vi "AMI MAG PHI IS_temp.vi"(0 "Y-Axis Communications Config":T3, 1 "delta H (mT)":dbl=0.5, 2 "delta phi (deg)":dbl=0.5, 3 "sweep parameter":T1=enum."magnetic field", 4 "const phi?":bool, 5 "Z-Axis Communications Config":T3, 7 "target mag in (T)":dbl, 9 "target phi (deg)":dbl, 11 "error in (no error)":T2) -> (6 "target mag out (T)":dbl[](array[numeric]), 8 "phi array (deg)":dbl[](array[numeric]), 15 "error out":T2)   [LabVIEW 2013]
uses:
  measurement/measurement sweep parameter.ctl
  <vilib>/Analysis/1siggen.llb/Ramp Pattern by Delta.vi
  <vilib>/Analysis/NI_AALBase.lvlib
panel:
  out "current mag (kG)":dbl
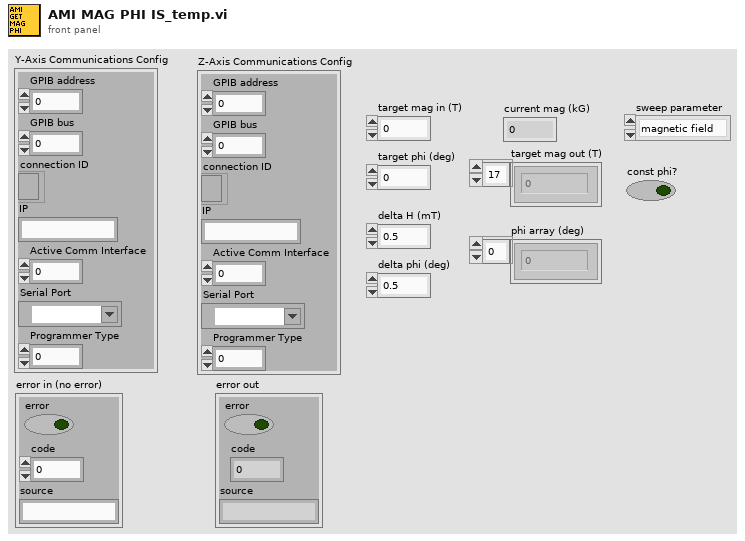
[diagram p1: front panel]
types:
  T1 = typedef "measurement sweep parameter.ctl" = enum16{"angle", "magnetic field"}
  T2 = cluster{"error":bool, "code":i32, "source":string}
  T3 = cluster{"GPIB address":i16, "GPIB bus":i16, "connection ID":refnum<k5>, "IP":string, "Active Comm Interface":u16, "Serial Port":refnum<visa-resource-name>, "Programmer Type":u16}
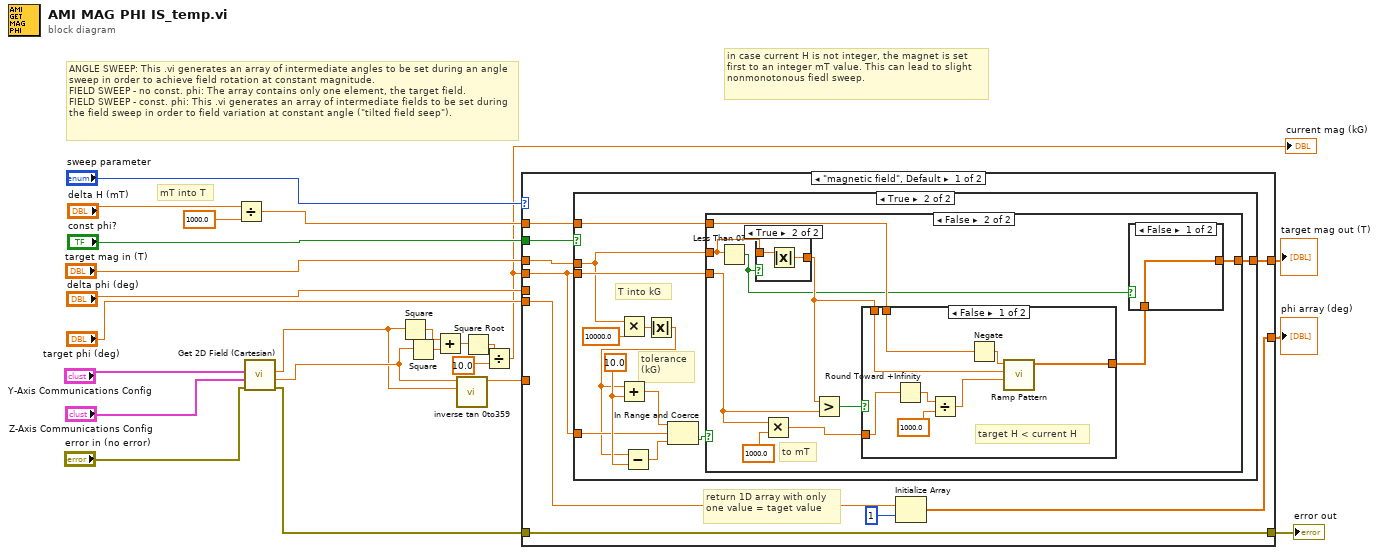
[diagram p0: block diagram]
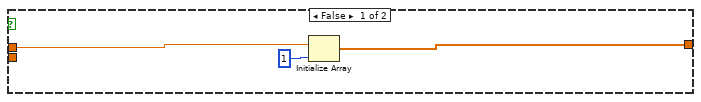
[diagram p2: hidden frame]
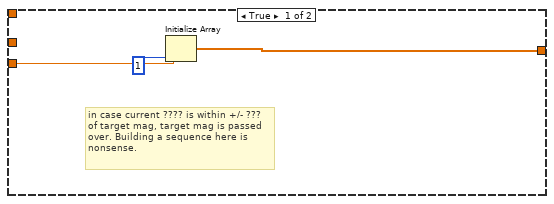
[diagram p3: hidden frame]
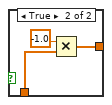
[diagram p4: hidden frame]
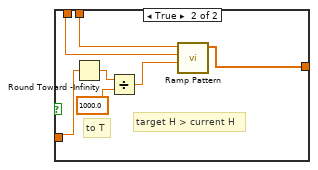
[diagram p6: hidden frame]
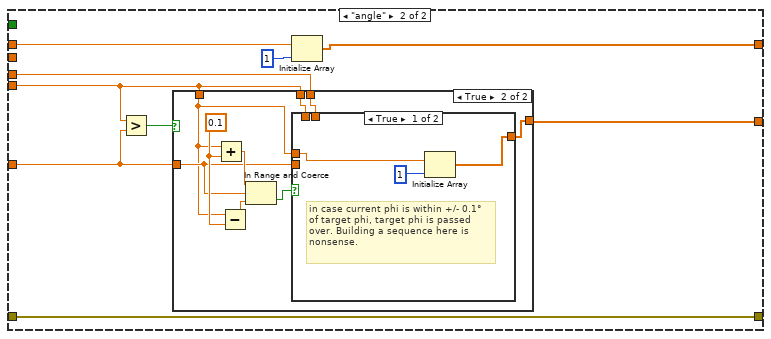
[diagram p7: hidden frame]
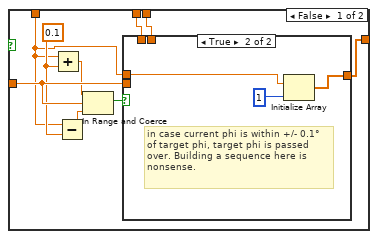
[diagram p8: hidden frame]
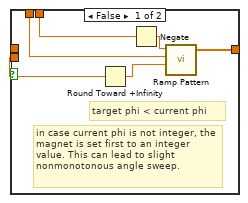
[diagram p9: hidden frame]
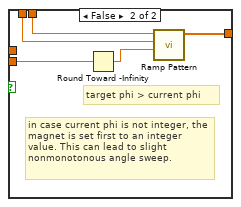
[diagram p10: hidden frame]
diagram:
  # "in case current H is not integer, the magnet is set first to an integer mT value. This can lead to slight nonmonotonous fiedl sweep."
  # "mT into T"
  # "ANGLE SWEEP: This .vi generates an array of intermediate angles to be set during an angle sweep in order to achieve field rotation at constant magnitude.\nFIELD SWEEP - no const. phi: The array contains only one element, the target field.\nFIELD SWEEP - const. phi: This .vi generates an array of intermediate fields to be set during the field sweep in order to field variation at constant angle (\"tilted field seep\")."
  n1 = Divide(x="delta H (mT)", y=1000.0) -> (x/y=w5:dbl)
  n2 = call <userlib>:"Get 2D Field (Cartesian).vi"("Y-Axis Communications Config"="Y-Axis Communications Config", "Z-Axis Communications Config"="Z-Axis Communications Config", "error in"="error in (no error)") -> ("Y-Axis Field (kG)"=w9:dbl, "Z-Axis Field (kG)"=w10:dbl, "error out"=w12:T2)  [unwired: 2 in, 1 out]
  n3 = Square(x=w9) -> (x^2=w20:dbl)
  n4 = Square(x=w10) -> (x^2=w19:dbl)
  n5 = Add(x=w20, y=w19) -> (x+y=w21:dbl)
  n6 = call "inverse tan 0to359.vi"("y coil"=w9, "z coil"=w10) -> ("phi (deg)"=w11:dbl)  [unwired: 9 in]
  n7 = Square Root(x=w21) -> (sqrt(x)=w1:dbl)
  n8 = Divide(x=w1, y=10.0) -> (x/y=w3:dbl)
  "current mag (kG)" <- w3
  n9 = case shown="\"magnetic field\", Default" "sweep parameter" {
    tunnel: "target phi (deg)" -> [w30 w84]
    tunnel: w11 -> [_ w88]
    tunnel: "delta phi (deg)" -> [_ w92]
    tunnel: [w31 w91] -> w16
    tunnel: [w28 w85] -> w8
    tunnel: "target mag in (T)" -> [w29 w86]
    tunnel: [w32 w90] -> w13
    tunnel: w12 -> [w32 w90]
    tunnel: "const phi?" -> [w27 _]
    tunnel: w3 -> [w25 _]
    tunnel: w5 -> [w26 _]
    frame "magnetic field", Default {
      # "return 1D array with only one value = taget value"
      n10 = case shown="True" w27 {
        tunnel: w29 -> [w35 w40]
        tunnel: [w34 w48] -> w28
        tunnel: w25 -> [_ w47]
        tunnel: w26 -> [_ w37]
        tunnel: w25 -> [_ w42]
        frame False {
          n11 = Initialize Array(w35, 1) -> (w34:dbl[])
        }
        frame True {
          w46 = 10.0
          # "tolerance (kG)"
          # "T into kG"
          n12 = Multiply(x=w40, y=10000.0) -> (x*y=w39:dbl)
          n13 = Absolute Value(x=w39) -> (abs(x)=w38:dbl)
          n14 = Add(x=w38, y=w46) -> (x+y=w44:dbl)
          n15 = Subtract(x=w38, y=w46) -> (x-y=w45:dbl)
          n16 = In Range and Coerce(upper limit=w44, x=w42, lower limit=w45) -> (In Range?=w43:bool)  [unwired: 1 out]
          n17 = case shown="False" w43 {
            tunnel: w40 -> [_ w55]
            tunnel: [w50 w52] -> w48
            tunnel: w47 -> [w49 w56]
            tunnel: w37 -> [_ w57]
            frame True {
              # "in case current ???? is within +/- ??? of target mag, target mag is passed over. Building a sequence here is nonsense."
              n18 = Initialize Array(w49, 1) -> (w50:dbl[])
            }
            frame False {
              # "to mT"
              n19 = Less Than 0?(x=w55) -> (x < 0?=w54:bool)
              n20 = case shown="True" w54 {
                tunnel: w55 -> [w66 w68]
                tunnel: [w66 w67] -> w58
                frame False {
                }
                frame True {
                  n21 = Absolute Value(x=w68) -> (abs(x)=w67:dbl)
                }
              }
              n22 = Multiply(x=w56, y=1000.0) -> (x*y=w60:dbl)
              n23 = Greater?(x=w58, y=w56) -> (0:w61:bool)
              n24 = case shown="False" w61 {
                tunnel: w58 -> [w74 w83]
                tunnel: w60 -> [w69 w77]
                tunnel: w57 -> [w75 w82]
                tunnel: [w73 w81] -> w53
                frame False {
                  # "target H < current H"
                  n25 = Round Toward +Infinity(x=w69) -> (ceil(x): smallest int >= x=w72:dbl)
                  n26 = Divide(x=w72, y=1000.0) -> (x/y=w70:dbl)
                  n27 = Negate(x=w75) -> (-x=w76:dbl)
                  n28 = call-poly <vilib>:"Ramp Pattern.vi"("start"=w70, "end"=w74, "delta"=w76) -> ("Ramp Pattern"=w73:dbl[])  [unwired: 6 in, 2 out]
                }
                frame True {
                  # "to T"
                  # "target H > current H"
                  n29 = Round Toward -Infinity(1:w77) -> (0:w80:dbl)
                  n30 = Divide(x=w80, y=1000.0) -> (x/y=w78:dbl)
                  n31 = call-poly <vilib>:"Ramp Pattern.vi"("start"=w78, "end"=w83, "delta"=w82) -> ("Ramp Pattern"=w81:dbl[])  [unwired: 6 in, 2 out]
                }
              }
              n32 = case shown="False" w54 {
                tunnel: w53 -> [w62 w64]
                tunnel: [w62 w63] -> w52
                frame False {
                }
                frame True {
                  n33 = Multiply(x=-1.0, y=w64) -> (x*y=w63:dbl[])
                }
              }
            }
          }
        }
      }
      n34 = Initialize Array(w30, 1) -> (w31:dbl[])
    }
    frame "angle" {
      n35 = Greater?(x=w84, y=w88) -> (0:w89:bool)
      n36 = case shown="True" w89 {
        tunnel: w84 -> [w100 w119]
        tunnel: w88 -> [w97 w112]
        tunnel: w92 -> [w101 w118]
        tunnel: [w99 w117] -> w91
        tunnel: w84 -> [w93 w111]
        frame False {
          w94 = 0.1
          n37 = Add(x=w93, y=w94) -> (x+y=w96:dbl)
          n38 = Subtract(x=w93, y=w94) -> (x-y=w95:dbl)
          n39 = In Range and Coerce(upper limit=w96, x=w97, lower limit=w95) -> (In Range?=w98:bool)  [unwired: 1 out]
          n40 = case shown="True" w98 {
            tunnel: w97 -> [w103 _]
            tunnel: w101 -> [w104 _]
            tunnel: w100 -> [w102 _]
            tunnel: [w105 w110] -> w99
            tunnel: w93 -> [_ w108]
            frame False {
              # "in case current phi is not integer, the magnet is set first to an integer value. This can lead to slight nonmonotonous angle sweep."
              # "target phi < current phi"
              n41 = Round Toward +Infinity(x=w103) -> (ceil(x): smallest int >= x=w107:dbl)
              n42 = Negate(x=w104) -> (-x=w106:dbl)
              n43 = call-poly <vilib>:"Ramp Pattern.vi"("start"=w107, "end"=w102, "delta"=w106) -> ("Ramp Pattern"=w105:dbl[])  [unwired: 6 in, 2 out]
            }
            frame True {
              # "in case current phi is within +/- 0.1° of target phi, target phi is passed over. Building a sequence here is nonsense."
              n44 = Initialize Array(w108, 1) -> (w110:dbl[])
            }
          }
        }
        frame True {
          w114 = 0.1
          n45 = Add(x=w111, y=w114) -> (x+y=w116:dbl)
          n46 = Subtract(x=w111, y=w114) -> (x-y=w115:dbl)
          n47 = In Range and Coerce(upper limit=w116, x=w112, lower limit=w115) -> (In Range?=w113:bool)  [unwired: 1 out]
          n48 = case shown="True" w113 {
            tunnel: w119 -> [_ w127]
            tunnel: w112 -> [_ w126]
            tunnel: w118 -> [_ w125]
            tunnel: [w121 w124] -> w117
            tunnel: w111 -> [w120 _]
            frame True {
              # "in case current phi is within +/- 0.1° of target phi, target phi is passed over. Building a sequence here is nonsense."
              n49 = Initialize Array(w120, 1) -> (w121:dbl[])
            }
            frame False {
              # "in case current phi is not integer, the magnet is set first to an integer value. This can lead to slight nonmonotonous angle sweep."
              # "target phi > current phi"
              n50 = Round Toward -Infinity(1:w126) -> (0:w123:dbl)
              n51 = call-poly <vilib>:"Ramp Pattern.vi"("start"=w123, "end"=w127, "delta"=w125) -> ("Ramp Pattern"=w124:dbl[])  [unwired: 6 in, 2 out]
            }
          }
        }
      }
      n52 = Initialize Array(w86, 1) -> (w85:dbl[])
    }
  }
  "error out" <- w13
  "phi array (deg)" <- w16
  "target mag out (T)" <- w8
